vi "TIFF-to-Fits.vi"() -> ()   [LabVIEW 2011]
uses:
  Library/tiff/TiffModules/ReadTiffPage_U16_text_res.vi
panel:
  out "read":i32
  out "error out":errorcluster
  in  "error in":errorcluster
  out "fits path":path
  in  "inputfile-Stack":path
  # "U16\nsorry needs lots of memory (whole dataset)"
  # "tut leider nicht so recht, großes tiff nicht komplett"
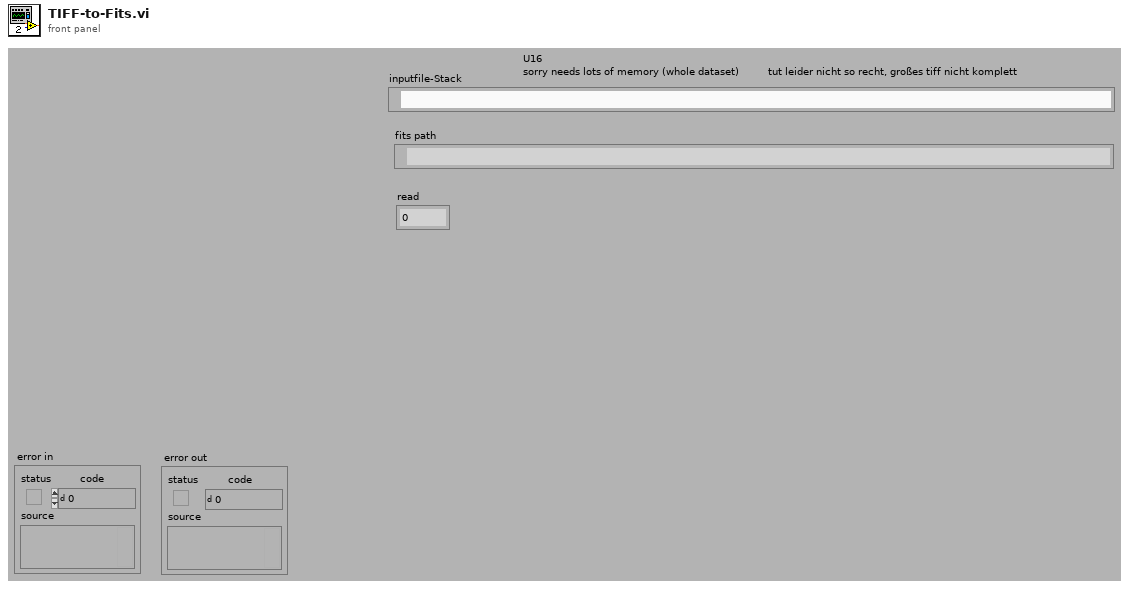
[diagram p1: front panel]
types:
  T1 = cluster{"Tiff refnum":refnum<file>, "BigTiff,Endian":u16}
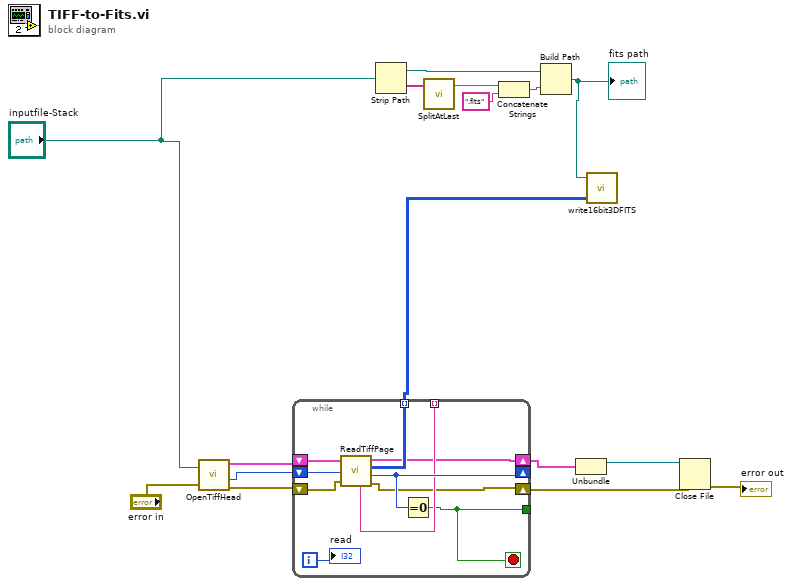
[diagram p0: block diagram]
diagram:
  n1 = call "OpenTiffHead.vi"("file path"="inputfile-Stack", "error in"="error in") -> ("TIFF file"=w8:T1, "first Diroffset"=w9:u64, "error out"=w7:errorcluster)  [unwired: 1 in]
  n2 = while {
    shift-right: [w23] -> _
    shift-left: w9 -> [w26]
    shift-right: [w19] -> w4
    shift-left: w8 -> [w25]
    shift-right: [w20] -> w3
    shift-left: w7 -> [w24]
    tunnel: [w18] -> _
    tunnel: [w22] -> w1 mode=indexing
    tunnel: [w21] -> _ mode=indexing
    i -> [w17]
    stop <- w18 stop-if-true
    n3 = call-poly "ReadTiffPage.vi"("TIFF file"=w25, "IFDoffset"=w26, "error in"=w24) -> ("TIFF file out"=w19:T1, "16-bit pixmap"=w22:u16[][], "string"=w21:string, "Next offset"=w23:i64, "error out"=w20:errorcluster)  [unwired: 2 in, 1 out]
    n4 = Equal To 0?(x=w23) -> (x = 0?=w18:bool)
    "read" <- w17
  }
  n5 = Strip Path(path="inputfile-Stack") -> (stripped path=w13:path, name=w14:string)
  n6 = call "SplitAtLast.vi"("In-String"=w14) -> ("Front (default)"=w15:string)  [unwired: 1 in, 1 out]
  n7 = Concatenate Strings(w15, ".fits" ("string")) -> (w16:string)
  n8 = Build Path(base path=w13, name or relative path=w16) -> (appended path=w11:path)
  "fits path" <- w11
  n9 = Unbundle(w4) -> ("Tiff refnum"=w6:refnum<file>)  [unwired: 1 out]
  n10 = call "write16bit3DFITS.vi"("u16 pixmap"=w1, "file path"=w11) -> ()  [unwired: 2 in, 1 out]
  n11 = Close File(refnum=w6, error in=w3) -> (error out=→"error out":errorcluster)  [unwired: 1 out]
